vi "RW Log File.vi"(8 "error in (no error)":errorcluster) -> (0 "error in (no error) 2":errorcluster)   [LabVIEW 2018]
uses:
  Log File/Log File.lvclass
  Log File/Log File.lvclass/Log File.ctl
  <vilib>/addons/_JKI Toolkits/Caraya/classes/Assert/Assert Equal Value_Variant.vi
  <vilib>/addons/_JKI Toolkits/Caraya/classes/Test/Test.lvclass
  <vilib>/addons/_JKI Toolkits/Caraya/classes/Assert/Assert.lvclass
panel:
  in  "file refnum":refnum<file>
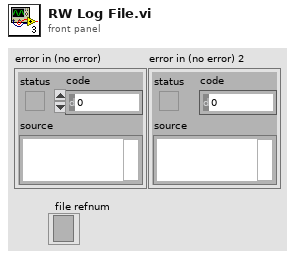
[diagram p1: front panel]
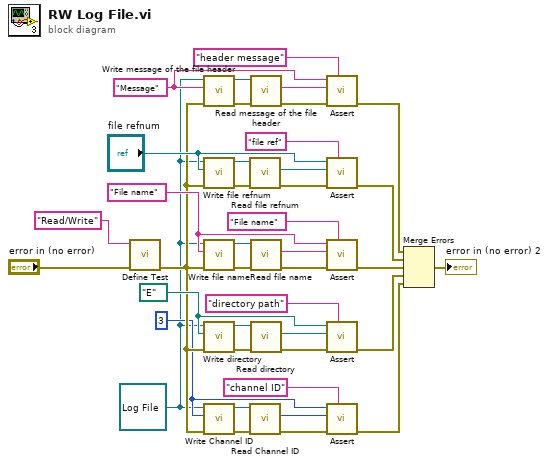
[diagram p0: block diagram]
diagram:
  w1 = refnum<class "Log File.lvclass"> refnum ("Log File.lvclass")
  w6 = u8 3 ("Channel ID")
  w15 = path "E:/" ("directory")
  w19 = "File name" ("file name")
  w34 = "Message" ("Label (VI Title)")
  n1 = call <vilib>:"Define Test.vi"("error in (no error)"="error in (no error)", "Label (VI Title)"="Read/Write") -> ("error out"=w8:errorcluster)  [unwired: 8 in, 1 out]
  n2 = call "Write message of the file header.vi"("error in (no error)"=w8, "message of the file header"=w34, "Log File in"=w1) -> ("error out"=w37:errorcluster, "Log File out"=w38:refnum<class "Log File.lvclass">)  [unwired: 7 in]
  n3 = call "Write file refnum.vi"("error in (no error)"=w8, "file refnum"="file refnum", "Log File in"=w1) -> ("error out"=w30:errorcluster, "Log File out"=w28:refnum<class "Log File.lvclass">)  [unwired: 7 in]
  n4 = call "Write file name.vi"("error in (no error)"=w8, "file name"=w19, "Log File in"=w1) -> ("error out"=w20:errorcluster, "Log File out"=w21:refnum<class "Log File.lvclass">)  [unwired: 7 in]
  n5 = call "Write directory.vi"("error in (no error)"=w8, "directory"=w15, "Log File in"=w1) -> ("error out"=w18:errorcluster, "Log File out"=w17:refnum<class "Log File.lvclass">)  [unwired: 7 in]
  n6 = call "Write Channel ID.vi"("error in (no error)"=w8, "Channel ID"=w6, "Log File in"=w1) -> ("error out"=w11:errorcluster, "Log File out"=w10:refnum<class "Log File.lvclass">)  [unwired: 7 in]
  n7 = call "Read file refnum.vi"("error in (no error)"=w30, "Log File in"=w28) -> ("error out"=w29:errorcluster, "file refnum"=w27:refnum<file>)  [unwired: 7 in, 1 out]
  n8 = call "Read Channel ID.vi"("error in (no error)"=w11, "Log File in"=w10) -> ("error out"=w9:errorcluster, "Channel ID"=w7:u8)  [unwired: 7 in, 1 out]
  n9 = call "Read message of the file header.vi"("error in (no error)"=w37, "Log File in"=w38) -> ("error out"=w36:errorcluster, "message of the file header"=w35:string)  [unwired: 7 in, 1 out]
  n10 = call "Read file name.vi"("error in (no error)"=w20, "Log File in"=w21) -> ("error out"=w23:errorcluster, "file name"=w22:string)  [unwired: 7 in, 1 out]
  n11 = call "Read directory.vi"("error in (no error)"=w18, "Log File in"=w17) -> ("error out"=w14:errorcluster, "directory"=w16:path)  [unwired: 7 in, 1 out]
  n12 = call-poly <vilib>:"Assert.vi"("Label"="header message", "error in (no error)"=w36, "Y"=w35, "X"=w34) -> ("error out"=w33:errorcluster)  [unwired: 6 in, 1 out]
  n13 = call-poly <vilib>:"Assert.vi"("Label"="file ref", "error in (no error)"=w29, "Y"=w27, "X"="file refnum") -> ("error out"=w25:errorcluster)  [unwired: 6 in, 1 out]
  n14 = call-poly <vilib>:"Assert.vi"("Label"="File name" ("file name"), "error in (no error)"=w23, "Y"=w22, "X"=w19) -> ("error out"=w4:errorcluster)  [unwired: 6 in, 1 out]
  n15 = call-poly <vilib>:"Assert.vi"("Label"="directory path" ("file name"), "error in (no error)"=w14, "Y"=w16, "X"=w15) -> ("error out"=w3:errorcluster)  [unwired: 6 in, 1 out]
  n16 = call-poly <vilib>:"Assert.vi"("Label"="channel ID" ("file name"), "error in (no error)"=w9, "Y"=w7, "X"=w6) -> ("error out"=w2:errorcluster)  [unwired: 6 in, 1 out]
  n17 = Merge Errors(w33, w25, w4, w3, w2) -> (→"error in (no error) 2":errorcluster)
